vi "RepairLine Array.vi"(10 "Array in":dbl[](array[numeric]), 11 "Index Array":dbl[](array[numeric])) -> (2 "Array Out":dbl[](array[numeric]))   [LabVIEW 2012]
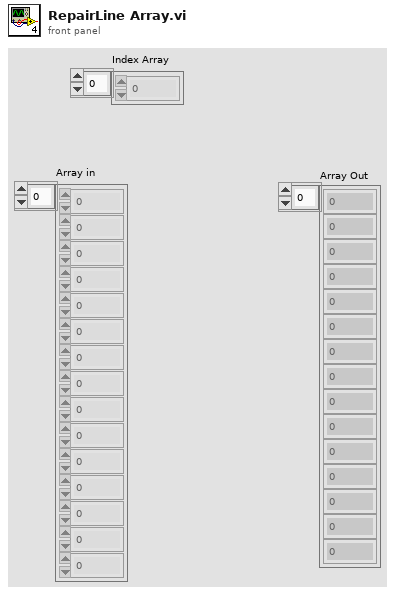
[diagram p1: front panel]
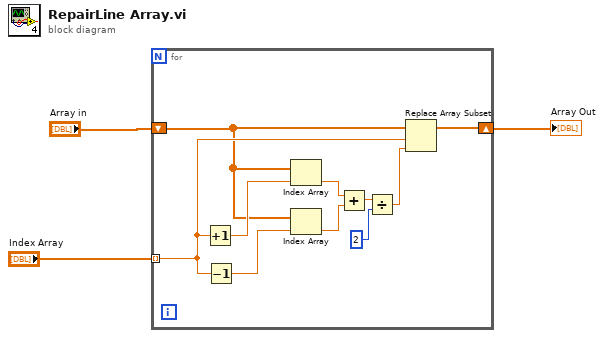
[diagram p0: block diagram]
diagram:
  n1 = for {
    tunnel: "Index Array" -> [w6] mode=indexing
    shift-right: [w5] -> w1
    shift-left: "Array in" -> [w4]
    n2 = Increment(x=w6) -> (x+1=w13:dbl)
    n3 = Decrement(x=w6) -> (x-1=w12:dbl)
    n4 = Index Array(array=w4, index=w13) -> (element=w11:dbl)
    n5 = Index Array(array=w4, index=w12) -> (element=w10:dbl)
    n6 = Add(x=w11, y=w10) -> (x+y=w9:dbl)
    n7 = Divide(x=w9, y=2) -> (x/y=w7:dbl)
    n8 = Replace Array Subset(array=w4, new element=w7, index=w6) -> (w5:dbl[])
  }
  "Array Out" <- w1
